vi "armPiston.vi"   [LabVIEW 2018]
uses:
  armPiston.ctl
  <vilib>/Rock Robotics/WPI/Solenoid/WPI_SolenoidValue.ctl
  <vilib>/Rock Robotics/WPI/Solenoid/WPI_SolenoidSetEnum.vi
types:
  T1 = typedef "WPI_SolenoidDevRef.ctl" = cluster{"DevStatus":errorcluster, "Pneumatics Control Module":u8, "Forward Solenoid Channel":T2, "Reverse Solenoid Channel":T2}
  T2 = typedef "WPI_SolenoidChannel.ctl" = enum8{"Solenoid 0", "Solenoid 1", "Solenoid 2", "Solenoid 3", "Solenoid 4", "Solenoid 5", "Solenoid 6", "Solenoid 7", "Invalid"}
  T3 = typedef "armPiston.ctl" = enum16{"out", "in"}
  T4 = typedef "WPI_SolenoidValue.ctl" = enum16{"Off", "On", "Forward", "Reverse"}
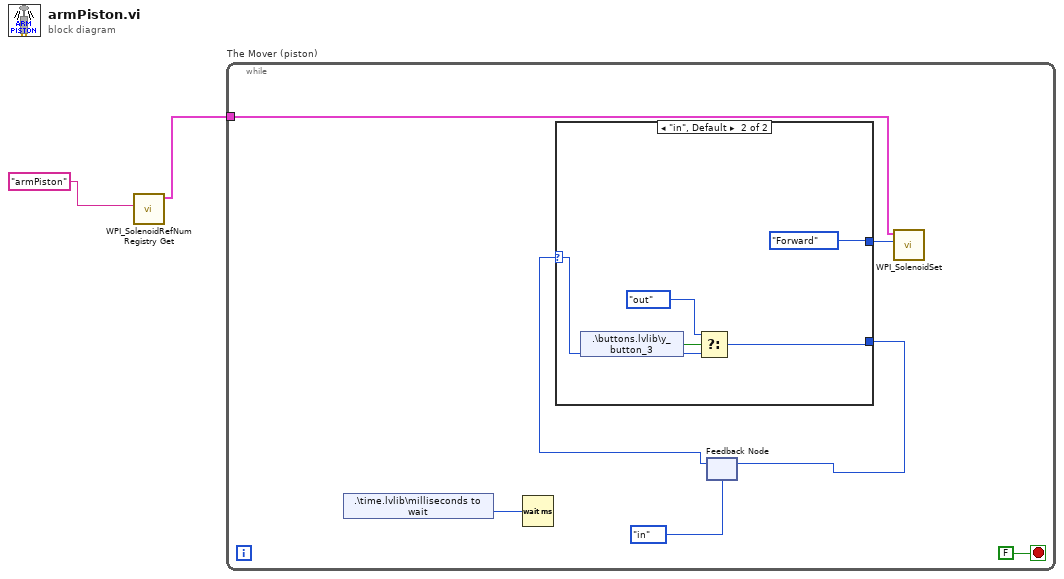
[diagram p0: block diagram]
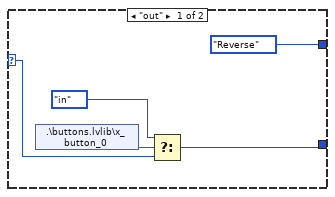
[diagram p2: hidden frame]
diagram:
  n1 = call <vilib>:"WPI_SolenoidRefNum Registry Get.vi"("refnum name"="armPiston") -> ("SolenoidDevRef"=w1:T1)  [unwired: 9 in, 1 out]
  n2 = while "The Mover (piston)" {
    tunnel: w1 -> [w3]
    stop <- FALSE stop-if-true
    n3 = shared-variable ".\\time.lvlib\\milliseconds to wait"() -> (w5:u32)  [unwired: 1 in, 1 out]
    n4 = Wait (ms)(milliseconds to wait=w5) -> ()  [unwired: 1 out]
    n5 = feedback #1(armPiston."in") -> (w8:T3)
    n6 = case shown="\"in\", Default" w8 {
      selector: w8 -> [w13 w18]
      tunnel: [w14 w19] -> w4
      tunnel: [WPI_SolenoidValue."Reverse" ("Value") WPI_SolenoidValue."Forward" ("Value")] -> w7
      frame "out" {
        n7 = shared-variable ".\\buttons.lvlib\\x_button_0"() -> (w10:bool)  [unwired: 1 in, 1 out]
        n8 = Select(t=armPiston."in", s=w10, f=w13) -> (s? t:f=w14:T3)
      }
      frame "in", Default {
        n9 = shared-variable ".\\buttons.lvlib\\y_button_3"() -> (w15:bool)  [unwired: 1 in, 1 out]
        n10 = Select(t=armPiston."out", s=w15, f=w18) -> (s? t:f=w19:T3)
      }
    }
    n11 = feedback-in #1(w4) -> ()
    n12 = call-poly <vilib>:"WPI_SolenoidSet.vi"("Value"=w7, "SolenoidDevRef"=w3) -> ()  [unwired: 8 in, 2 out]
  }
